vi "Aim With Position.vi"() -> (0 "Aimpoint Distance (ft)":dbl, 2 "Target Gyro Angle":dbl, 10 "Aimpoint X-Coord":dbl)   [LabVIEW 2013]
uses:
  Robot Global Data.vi
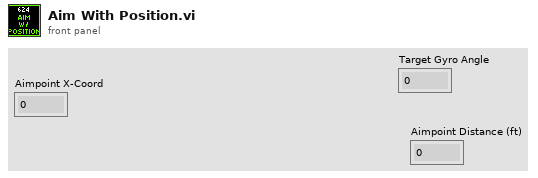
[diagram p1: front panel]
types:
  T1 = typedef "Shooter Manual Control.ctl" = cluster{"Command":T2, "Offset":dbl, "Trigger":bool, "Add":bool, "Release":bool, "Reset":bool, "Target Pressure":dbl}
  T2 = typedef "Shooter Command.ctl" = enum16{"None", "Warmup", "Shoot"}
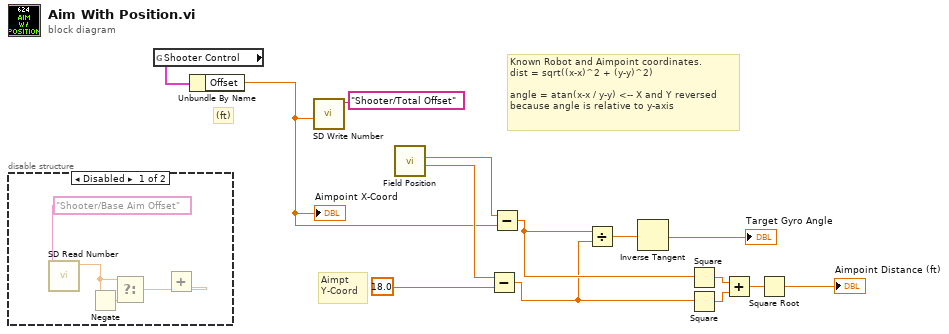
[diagram p0: block diagram]
diagram:
  # "(ft)"
  # "Known Robot and Aimpoint coordinates.\ndist = sqrt((x-x)^2 + (y-y)^2)\n\nangle = atan(x-x / y-y) <-- X and Y reversed\nbecause angle is relative to y-axis"
  # "Aimpt \nY-Coord"
  n1 = disable-structure shown="Disabled" {
    frame Disabled {
      n2 = call <vilib>:"SD Read Number.vi"("Name"="Shooter/Base Aim Offset") -> ("Numeric"=w16:dbl)  [unwired: 8 in, 2 out]
      n3 = Negate(x=w16) -> (-x=w17:dbl)
      n4 = Select(t=w16, f=w17) -> (s? t:f=w15:dbl)  [unwired: 1 in]
      n5 = Add(y=w15) -> ()  [unwired: 1 in, 1 out]
    }
    frame Enabled {
    }
  }
  n6 = global read "Robot Global Data.vi" "Shooter Control"() -> (w2:T1)
  n7 = Unbundle By Name(w2) -> ("Offset"=w1:dbl)
  "Aimpoint X-Coord" <- w1
  n8 = call <vilib>:"SD Write Number.vi"("Numeric"=w1, "Name"="Shooter/Total Offset") -> ()  [unwired: 8 in, 2 out]
  n9 = call "Field Position.vi"() -> ("Field Y"=w13:dbl, "Field X"=w14:dbl)  [unwired: 9 in, 1 out]
  n10 = Subtract(x=w13, y=18.0) -> (x-y=w6:dbl)
  n11 = Subtract(x=w14, y=w1) -> (x-y=w7:dbl)
  n12 = Divide(x=w7, y=w6) -> (x/y=w5:dbl)
  n13 = Inverse Tangent(1:w5) -> (0:→"Target Gyro Angle":dbl)
  n14 = Square(x=w7) -> (x^2=w11:dbl)
  n15 = Square(x=w6) -> (x^2=w10:dbl)
  n16 = Add(x=w11, y=w10) -> (x+y=w9:dbl)
  n17 = Square Root(x=w9) -> (sqrt(x)=→"Aimpoint Distance (ft)":dbl)
